vi "Save.vi"(8 "error in (no error)":errorcluster, 9 "new command":string, 10 "Msg in":T1, 11 "MagSpec_Bella in":refnum<class "MagSpec_Bella.lvclass">) -> (0 "error out":errorcluster, 1 "Path":path, 2 "Msg out":T1, 3 "MagSpec_Bella out":refnum<class "MagSpec_Bella.lvclass">, 4 "new command":string)   [LabVIEW 2020, in "MagSpec_Bella.lvclass"]
uses:
  MagSpec_Bella.lvclass
  DriverMsg.ctl
  C:/GEECS/Developers Version/source/Device Drivers/BaseDriver/BaseDriver.lvclass
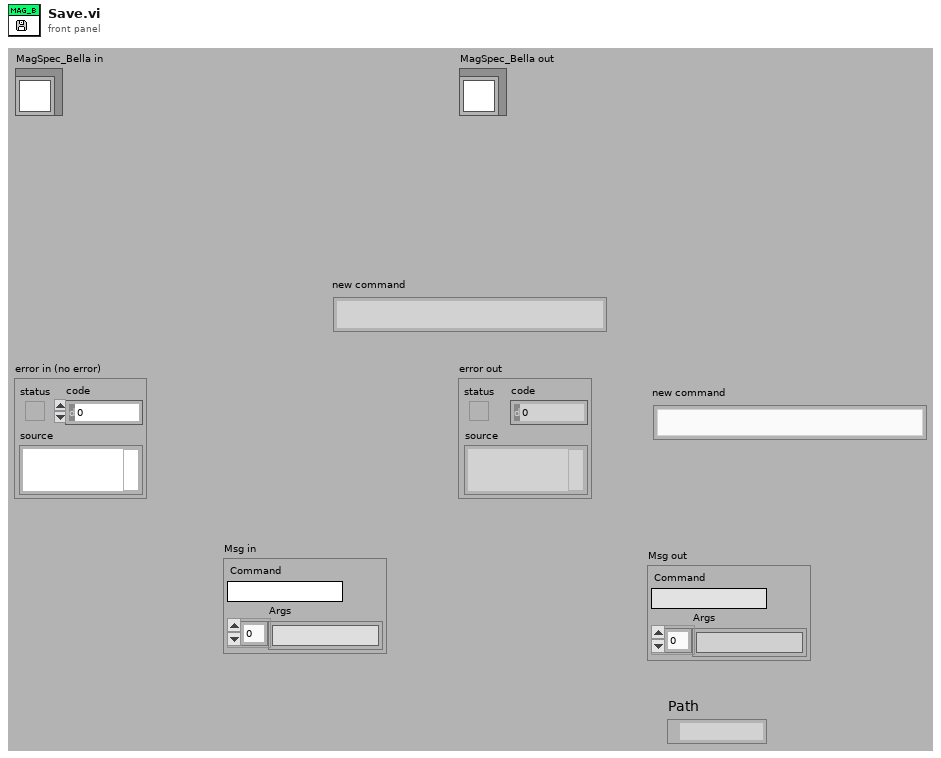
[diagram p1: front panel]
types:
  T1 = typedef "DriverMsg.ctl" = cluster{"Command":string, "Args":string[]}
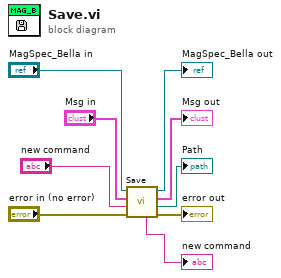
[diagram p0: block diagram]
diagram:
  n1 = call-parent "Save.vi"("error in (no error)"="error in (no error)", "new command"="new command", "Msg in"="Msg in", "BaseDriver in"="MagSpec_Bella in") -> ("error out"=→"error out":errorcluster, "Path"=→"Path":path, "Msg out"=→"Msg out":T1, "BaseDriver out"=→"MagSpec_Bella out":refnum<class "MagSpec_Bella.lvclass">, "new command"=→"new command":string)  [unwired: 3 in]
